vi "opgave 3.3.vi"() -> ()   [LabVIEW 2015]
panel:
  out "Waveform Chart":cluster{"number: 0 to 1":dbl, dbl}(graph)
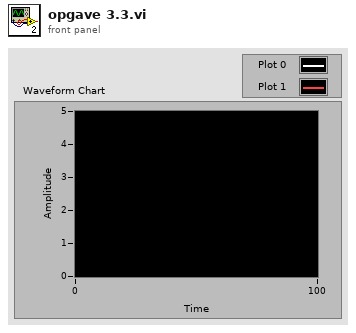
[diagram p1: front panel]
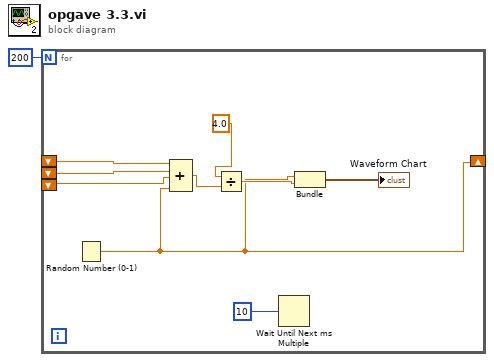
[diagram p0: block diagram]
diagram:
  n1 = for {
    N: 200 -> [_]
    shift-right: [w4] -> _
    shift-left: _ -> [w10]
    shift-left: _ -> [w6]
    shift-left: _ -> [w2]
    n2 = Random Number (0-1)() -> (number: 0 to 1=w4:dbl)
    n3 = Compound Arithmetic op=ADD(w10, w6, w2, w4) -> (w9:dbl)
    n4 = Divide(x=4.0, y=w9) -> (x/y=w7:dbl)
    n5 = Wait Until Next ms Multiple(millisecond multiple=10) -> ()  [unwired: 1 out]
    n6 = Bundle("number: 0 to 1"=w4, w7) -> (→"Waveform Chart":cluster{"number: 0 to 1":dbl, dbl})  [unwired: 1 in]
  }
